vi "Add Children to Tree.vi"(8 "error in (no error)":errorcluster, 9 "Parent Tag":string, 10 "Tree Manager in":refnum<class "Tree Manager.lvclass">, 11 "Data Item in":refnum<class "Data Item.lvclass">) -> (0 "error out":errorcluster, 2 "Tree Manager out":refnum<class "Tree Manager.lvclass">, 3 "Data Item out":refnum<class "Data Item.lvclass">)   [LabVIEW 2023, in "VILab.lvlib" / "Data Item.lvclass"]
uses:
  Data Item.lvclass
  Tree Manager/Tree Manager.lvclass
  Data Item.lvclass/Data Item.ctl
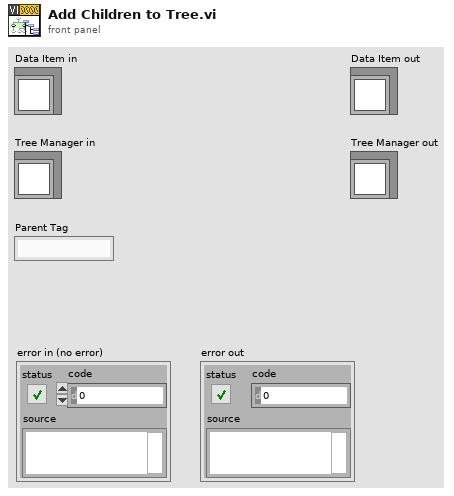
[diagram p1: front panel]
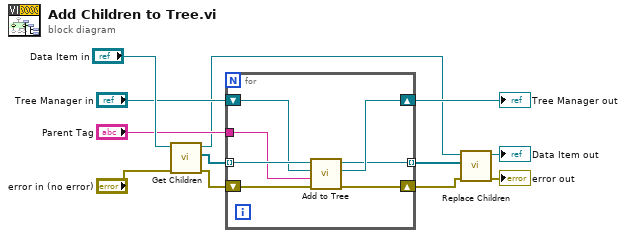
[diagram p0: block diagram]
diagram:
  n1 = call-dynamic "Get Children.vi"("error in (no error)"="error in (no error)", "Data Item in"="Data Item in") -> ("error out"=w11:errorcluster, "Children"=w12:refnum<class "Data Item.lvclass">[], "Data Item out"=w1:refnum<class "Data Item.lvclass">)  [unwired: 7 in]
  n2 = for {
    shift-right: [w15] -> w4
    shift-left: "Tree Manager in" -> [w18]
    shift-right: [w16] -> w7
    shift-left: w11 -> [w17]
    tunnel: w12 -> [w19] mode=indexing
    tunnel: "Parent Tag" -> [w14]
    tunnel: [w13] -> w5 mode=indexing
    n3 = call-dynamic "Add to Tree.vi"("error in (no error)"=w17, "Parent Tag"=w14, "Tree Manager in"=w18, "Data Item in"=w19) -> ("error out"=w16:errorcluster, "Tree Manager out"=w15:refnum<class "Tree Manager.lvclass">, "Data Item out"=w13:refnum<class "Data Item.lvclass">)  [unwired: 5 in]
  }
  "Tree Manager out" <- w4
  n4 = call-dynamic "Replace Children.vi"("error in (no error)"=w7, "New Children"=w5, "Data Item in"=w1) -> ("error out"=→"error out":errorcluster, "Data Item out"=→"Data Item out":refnum<class "Data Item.lvclass">)  [unwired: 7 in]
